vi "VIP_Post-Install Custom Action.vi"(10 "Variant":variant) -> (0 "error out":errorcluster)   [LabVIEW 2021]
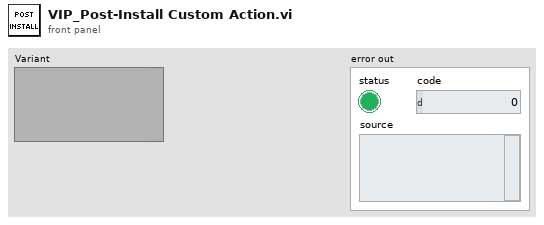
[diagram p1: front panel]
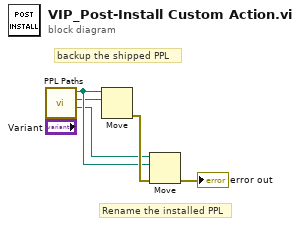
[diagram p0: block diagram]
diagram:
  # "Rename the installed PPL"
  # "backup the shipped PPL"
  n1 = call "PPL Paths.vi"() -> ("Install PPL"=w1:path, "Shipped Backup"=w2:path, "Current PPL"=w3:path)  [unwired: 9 in]
  n2 = Move(source path=w3, 10:w2) -> (error out=w5:errorcluster)  [unwired: 3 in, 2 out]
  n3 = Move(source path=w1, error in=w5, 10:w3) -> (error out=→"error out":errorcluster)  [unwired: 2 in, 2 out]
